vi "Read t0.vi"(8 "error in (no error)":errorcluster, 11 "Start Stream Result in":refnum<class "Start Stream Result.lvclass">) -> (0 "error out":errorcluster, 2 "t0":dbl, 3 "Start Stream Result out":refnum<class "Start Stream Result.lvclass">)   [LabVIEW 2019, in "Start Stream Result.lvclass"]
uses:
  Start Stream Result.lvclass
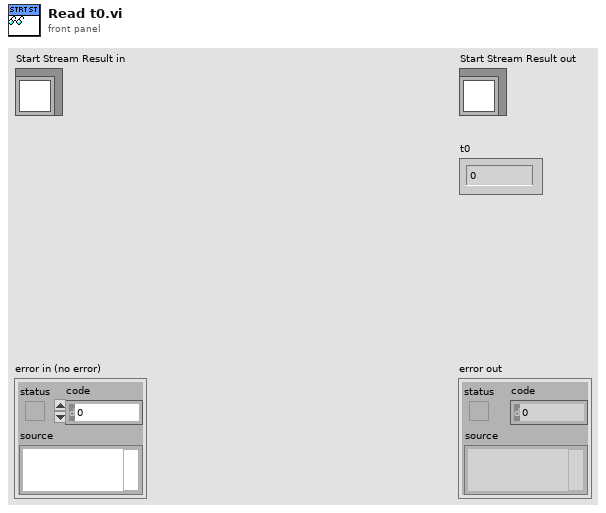
[diagram p1: front panel]
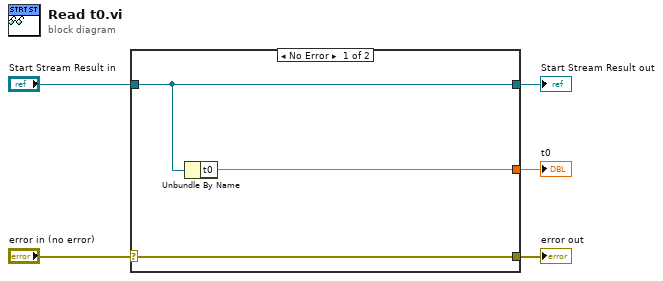
[diagram p0: block diagram]
diagram:
  n1 = case shown="No Error" "error in (no error)" {
    selector: "error in (no error)" -> [w8 w9]
    tunnel: [w8 w9] -> w4
    tunnel: [w7 w10] -> w2
    tunnel: "Start Stream Result in" -> [w7 w10]
    tunnel: [w6 _] -> w1
    frame No Error {
      n2 = Unbundle By Name(w7) -> ("t0"=w6:dbl)
    }
    frame Error {
    }
  }
  "error out" <- w4
  "Start Stream Result out" <- w2
  "t0" <- w1
